vi "Write Command.vi"(8 "error in (no error)":errorcluster, 9 "Responses in":T1[](array[typedef]) {"Command" items=["Constant Speed Tracking"=8, "Echo"=55, "Error"=255, "Home"=1, "Limit Active"=9, "Manual Move Tracking"=10, "Move Absolute"=20, "Move at Constant Speed"=22, "Move Relative"=21, "Renumber"=2, "Restore Settings"=36, "Stop"=23]}, 10 "Request":T2={"Device Number"=0, "Command"=0, "Data"=0, "Response Count"=1} {"Command" items=["Echo"=55, "Home"=1, "Move Absolute"=20, "Move Relative"=21, "Move at Constant Speed"=22, "Renumber"=2, "Restore Settings"=36, "Stop"=23]}, 11 "VISA resource name":refnum<visa-resource-name>) -> (0 "error out":errorcluster, 1 "Responses out":T1[](array[typedef]) {"Command" items=["Constant Speed Tracking"=8, "Echo"=55, "Error"=255, "Home"=1, "Limit Active"=9, "Manual Move Tracking"=10, "Move Absolute"=20, "Move at Constant Speed"=22, "Move Relative"=21, "Renumber"=2, "Restore Settings"=36, "Stop"=23]}, 3 "VISA resource name out":refnum<visa-resource-name>)   [LabVIEW 2013, in "ZaberTSeries.lvlib"]
doc: "Writes a command to a Zaber device through the serial port."
uses:
  ZaberTSeries.lvlib
  Utility/Request.ctl
  Utility/Response.ctl
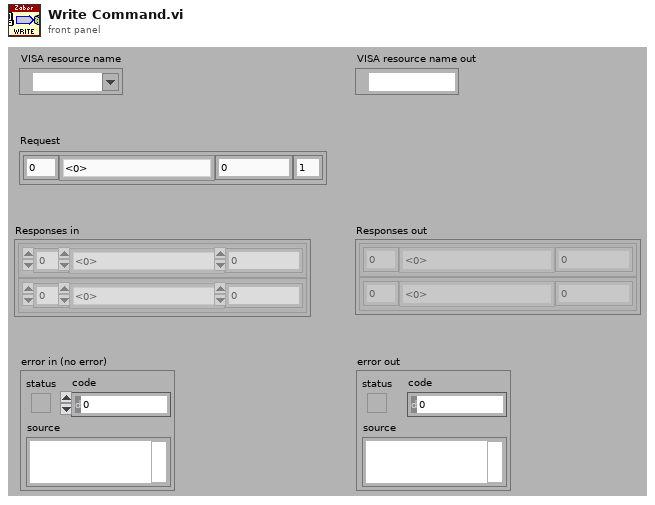
[diagram p1: front panel]
types:
  T1 = typedef "ZaberTSeries.lvlib/Response.ctl" = cluster{"Device Number":u8, "Command":u8, "Data":i32}
  T2 = typedef "ZaberTSeries.lvlib/Request.ctl" = cluster{"Device Number":u8, "Command":u8, "Data":i32, "Response Count":i32}
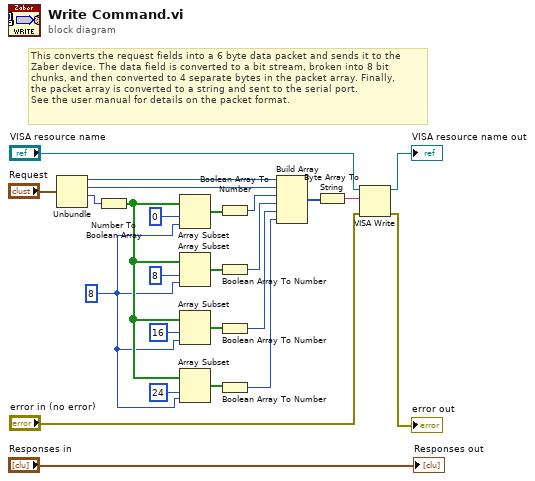
[diagram p0: block diagram]
diagram:
  w11 = 8 ("length")
  # "This converts the request fields into a 6 byte data packet and sends it to the\nZaber device. The data field is converted to a bit stream, broken into 8 bit\nchunks, and then converted to 4 separate bytes in the packet array. Finally,\nthe packet array is converted to a string and sent to the serial port.\nSee the user manual for details on the packet format."
  n1 = Unbundle("Request") -> ("Device Number"=w6:u8, "Command"=w5:u8, "Data"=w4:i32)  [unwired: 1 out]
  n2 = Number To Boolean Array(number=w4) -> (Boolean array=w13:bool[])
  n3 = Array Subset(array=w13, index=0, length=w11) -> (w21:bool[])
  n4 = Array Subset(array=w13, index=8, length=w11) -> (w16:bool[])
  n5 = Array Subset(array=w13, index=16, length=w11) -> (w14:bool[])
  n6 = Array Subset(array=w13, index=24, length=w11) -> (w10:bool[])
  n7 = Boolean Array To Number(Boolean array=w21) -> (number=w20:u32)
  n8 = Boolean Array To Number(Boolean array=w16) -> (number=w15:u32)
  n9 = Boolean Array To Number(Boolean array=w14) -> (number=w8:u32)
  n10 = Boolean Array To Number(Boolean array=w10) -> (number=w9:u32)
  n11 = Build Array(w6, w5, w20, w15, w8, w9) -> (w24:u32[])
  n12 = Byte Array To String(unsigned byte array=w24) -> (string=w25:string)
  n13 = VISA Write(VISA resource name="VISA resource name", write buffer=w25, error in (no error)="error in (no error)") -> (VISA resource name out=→"VISA resource name out":refnum<visa-resource-name>, error out=→"error out":errorcluster)  [unwired: 1 out]
  "Responses out" <- "Responses in"
